vi "Authenticate.vi"(8 "error in (no error)":errorcluster, 10 "Challenge Dict":string, 11 "IAuthenticator in":refnum<class "IAuthenticator.lvclass">) -> (0 "error out":errorcluster, 1 "Authenticate Dict":string, 2 "Authenticate Signature":string, 3 "IAuthenticator out":refnum<class "IAuthenticator.lvclass">)   [LabVIEW 2020, in "wamplv.lvlib" / "IAuthenticator.lvclass"]
uses:
  IAuthenticator.lvclass
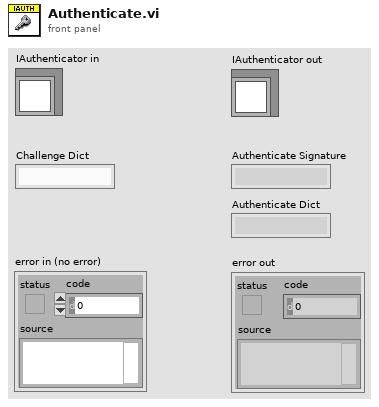
[diagram p1: front panel]
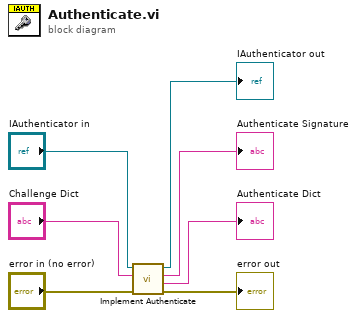
[diagram p0: block diagram]
diagram:
  n1 = call-dynamic "Implement Authenticate.vi"("error in (no error)"="error in (no error)", "Challenge Dict"="Challenge Dict", "IAuthenticator in"="IAuthenticator in") -> ("error out"=→"error out":errorcluster, "Authenticate Dict"=→"Authenticate Dict":string, "Authenticate Signature"=→"Authenticate Signature":string, "IAuthenticator out"=→"IAuthenticator out":refnum<class "IAuthenticator.lvclass">)  [unwired: 5 in]
